vi "Reactive Power.vi"(4 "Active Power":dbl, 5 "Apparent Power":dbl) -> (1 "Reactive Power":dbl)   [LabVIEW 2014]
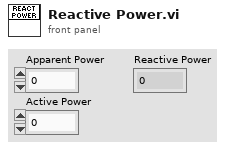
[diagram p1: front panel]
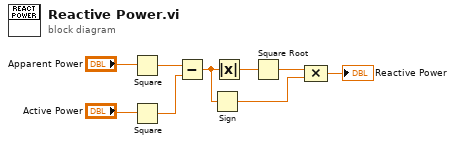
[diagram p0: block diagram]
diagram:
  n1 = Square(x="Apparent Power") -> (x^2=w9:dbl)
  n2 = Square(x="Active Power") -> (x^2=w8:dbl)
  n3 = Subtract(x=w9, y=w8) -> (x-y=w4:dbl)
  n4 = Sign(1:w4) -> (0:w2:dbl)
  n5 = Absolute Value(x=w4) -> (abs(x)=w5:dbl)
  n6 = Square Root(x=w5) -> (sqrt(x)=w3:dbl)
  n7 = Compound Arithmetic op=MULTIPLY(w3, w2) -> (→"Reactive Power":dbl)
